vi "Test Method 1.vi"(11 "Test Case In":refnum<class "My Test Case.lvclass">) -> (0 "error out":errorcluster, 3 "Test Case Out":refnum<class "My Test Case.lvclass">)   [LabVIEW 2020, in "My Test Case.lvclass"]
uses:
  My Test Case.lvclass
  C:/Program Files (x86)/National Instruments/LabVIEW 2020/vi.lib/Astemes/LUnit/Test Case.lvclass
  <vilib>/Astemes/LUnit/Test Case.lvclass/Test Case.ctl
  4993e8ee-a06a-463a-9684-69129f64d5ce.vi
  <vilib>/Astemes/LUnit/Core/LUnit Test Case/Private/Append Pass Result.vi
  <vilib>/Astemes/LUnit/Core/LUnit Test Case/Private/Append Fail Result.vi
  4993e8ee-a06a-463a-9684-69129f64d5ce.vi/9c5d11cd-9439-4240-a1ee-d9baace9c924.vi
  <vilib>/Astemes/LUnit/Core/LUnit Test Case/Private/Run In UI.vi
  <vilib>/Utility/error.llb/Clear Errors.vi
  My Test Case.lvclass/My Test Case.ctl
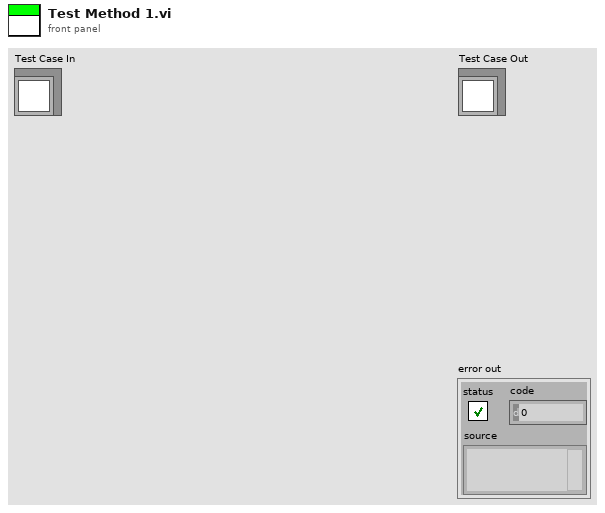
[diagram p1: front panel]
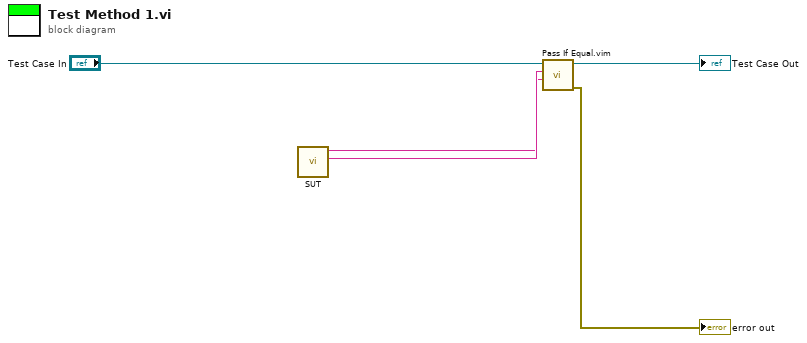
[diagram p0: block diagram]
diagram:
  n1 = call "SUT.vi"() -> ("String 2"=w2:string, "String"=w1:string)  [unwired: 10 in]
  n2 = call "Pass If Equal.vim"("Actual"=w1, "Expected"=w2, "LUnit Test Case In"="Test Case In") -> ("error out"=→"error out":errorcluster, "LUnit Test Case Out"=→"Test Case Out":refnum<class "My Test Case.lvclass">)  [unwired: 7 in]
